vi "change table color.vi"(11 "MulticolumnListbox输入":refnum<vi>) -> ()   [LabVIEW 2016]
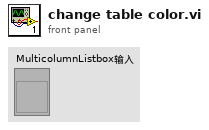
[diagram p1: front panel]
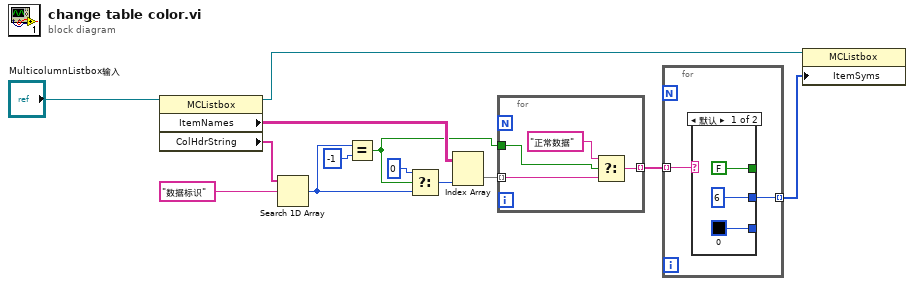
[diagram p0: block diagram]
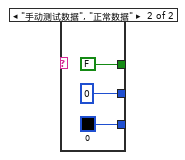
[diagram p2: hidden frame]
diagram:
  n1 = property class="MCListbox"(reference="MulticolumnListbox输入") -> (reference out=w1:refnum<vi>, "ItemNames"=w13:string[][], "ColHdrString"=w11:string[])  [unwired: 1 in, 1 out]
  n2 = Search 1D Array(1D array=w11, element="数据标识" ("元素")) -> (index of element=w8:i32)  [unwired: 1 in]
  n3 = Equal?(x=w8, y=-1) -> (x = y?=w4:bool)
  n4 = Select(t=0, s=w4, f=w8) -> (s? t:f=w6:i32)
  n5 = Index Array(array=w13, index (col)=w6) -> (element=w5:string[])  [unwired: 1 in]
  n6 = for {
    tunnel: w5 -> [w15] mode=indexing
    tunnel: w4 -> [w17]
    tunnel: [w14] -> w3 mode=indexing
    n7 = Select(t="正常数据", s=w17, f=w15) -> (s? t:f=w14:string)
  }
  n8 = for {
    tunnel: w3 -> [w19] mode=indexing
    tunnel: [w18] -> w2 mode=indexing
    n9 = case shown="默认" w19 {
      tunnel: [FALSE FALSE] -> _
      tunnel: [u32 0 u32 0] -> _
      tunnel: [6 0] -> w18
      frame Default {
      }
      frame "手动测试数据", "正常数据" {
      }
    }
  }
  n10 = property class="MCListbox"(reference=w1, "ItemSyms"=w2) -> ()  [unwired: 1 in, 2 out]
